vi "myo_imu_data.vi"() -> ()   [LabVIEW 2013]
uses:
  <vilib>/BLE/type_def/address_type.ctl
  type_def/unlock_types.ctl
  type_def/emg_mode.ctl
  type_def/imu_mode.ctl
  <vilib>/BLE/type_def/connection_status_bundle.ctl
panel:
  out "full message package 2":u8[](array[numeric]) format="%02x"
  out "Unlock?":bool
  out "Numeric":i32
  out "full message package":u8[][](array[numeric]) format="%02x"
  out "Battery?":bool
  out "Handler Table?":bool
  out "Connected?":bool
  out "Tank":dbl(slide) scale=0.0..100.0
  in  "stop":bool
  out "MYO Handler Table":string[][](array[string])
  out "Connection Status":T1={"MAC Address"="", "cnx handle"=0, "cnx flags"=0, "Address Type"=125, "Connection Interval (ms)"=125, "Timeout(ms)"=125, "Latency"=0, "bonding handle"=0} {"Address Type" items=["Public", "Random"]}
  in  "COM Bluegiga in":refnum<visa-resource-name>="COM13"
  out "BLED112 Dongle Info":string
  # "DONGLE"
  # "READING"
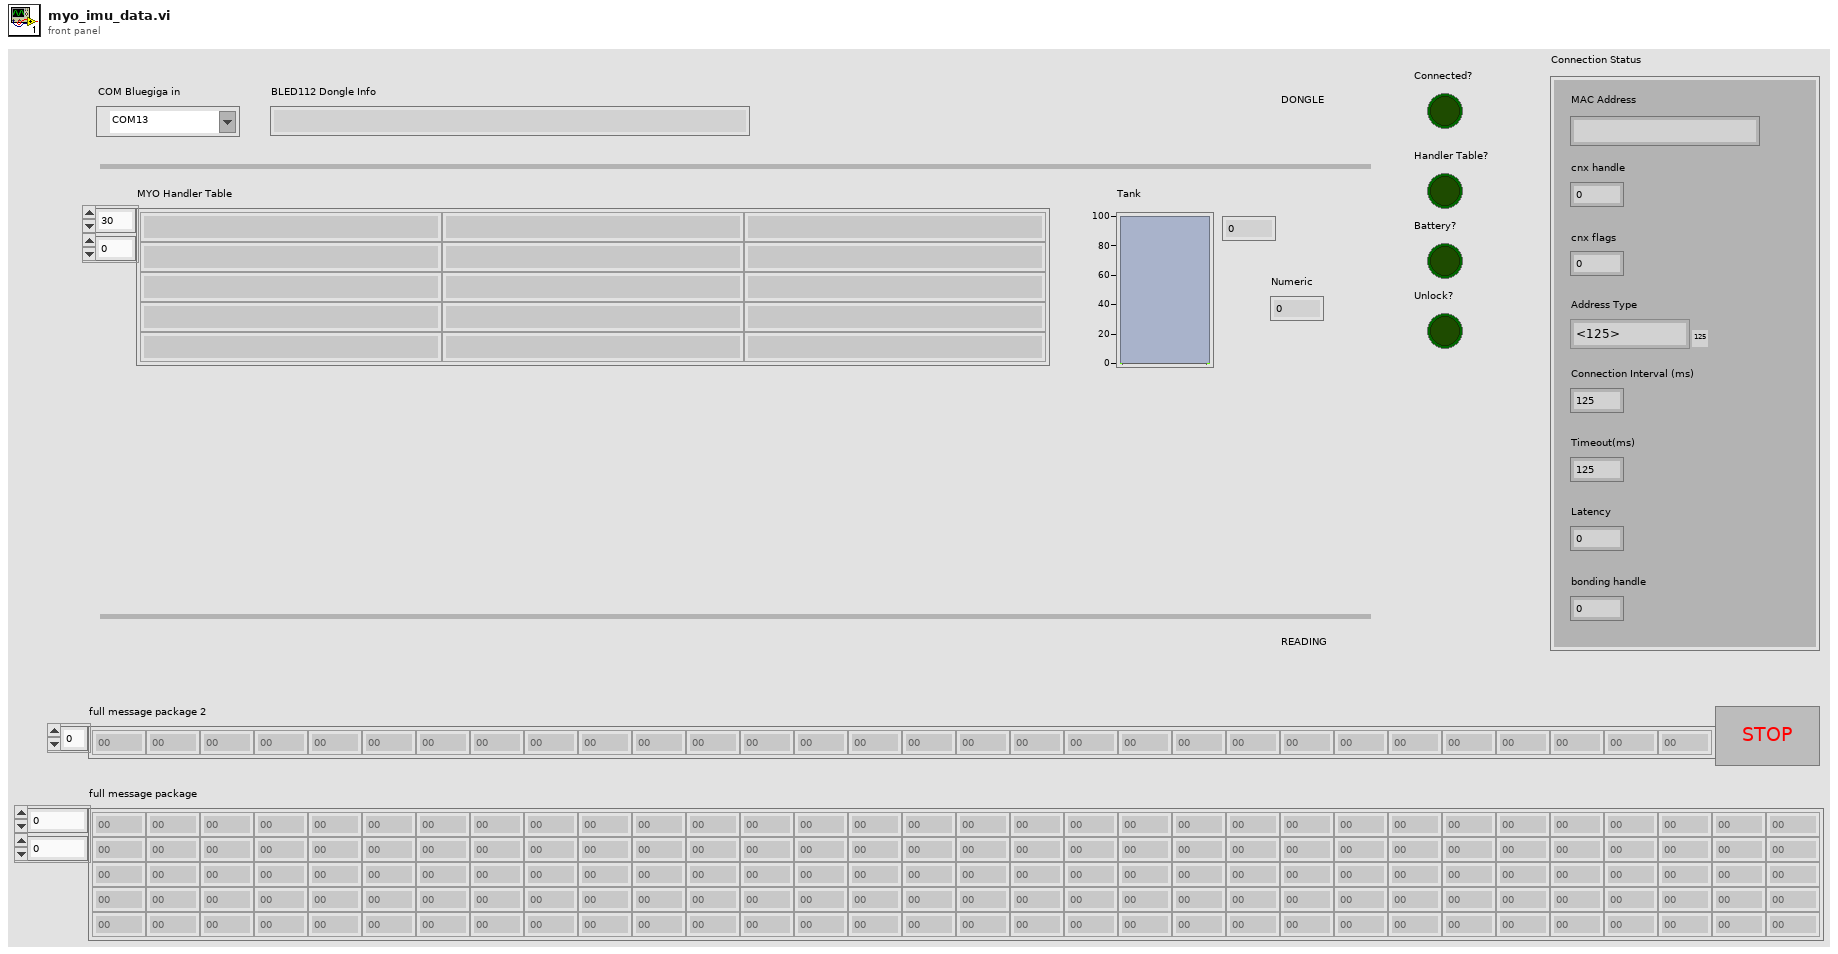
[diagram p1: front panel]
types:
  T1 = typedef "connection_status_bundle.ctl" = cluster{"MAC Address":string, "cnx handle":u8, "cnx flags":u8, "Address Type":T2, "Connection Interval (ms)":u16, "Timeout(ms)":u16, "Latency":u16, "bonding handle":u8}
  T2 = typedef "address_type.ctl" = u8
  T3 = typedef "imu_mode.ctl" = u8
  T4 = typedef "emg_mode.ctl" = u8
  T5 = typedef "unlock_types.ctl" = u8
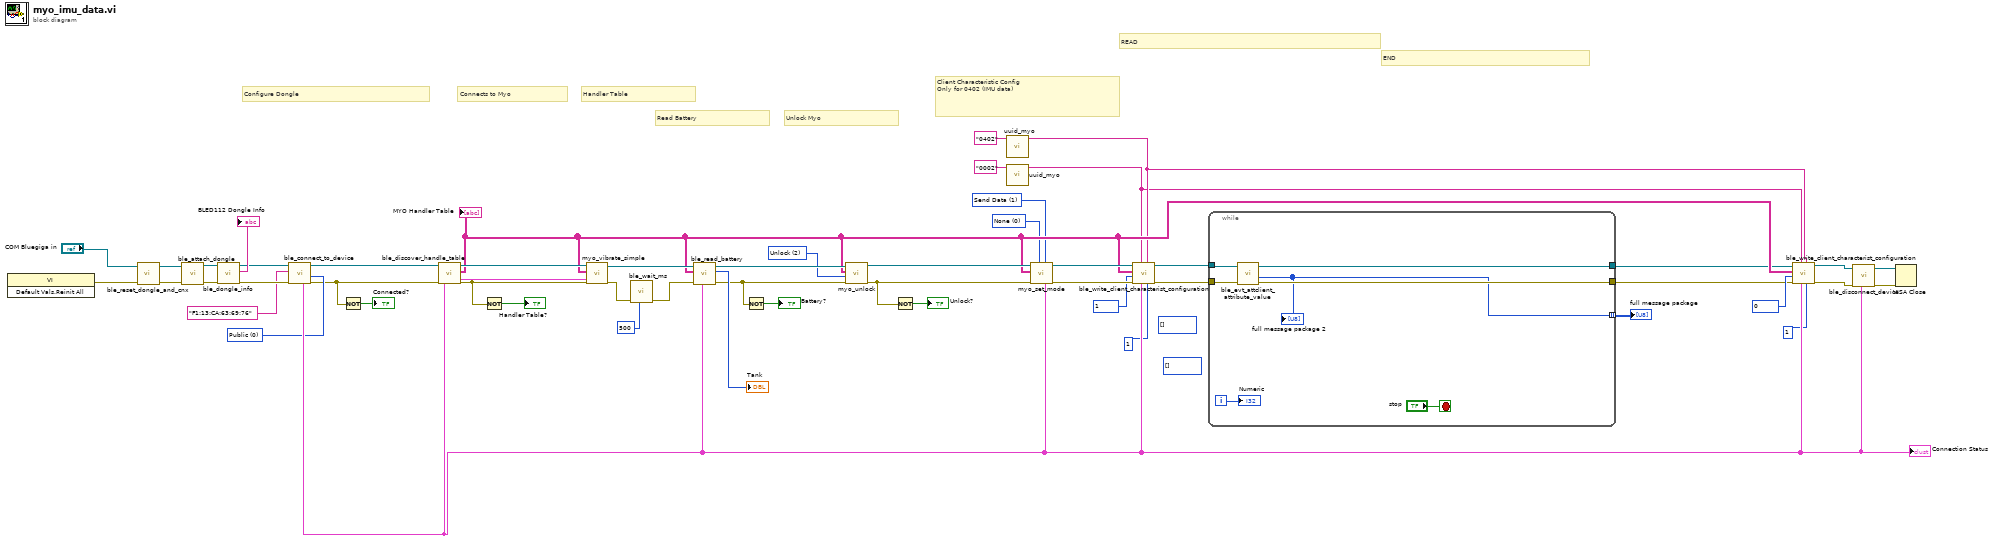
[diagram p0: block diagram]
diagram:
  w2 = T3 1 items=["None", "Send Data", "Send Events", "Send All", "Send Raw"] ("IMU mode (None)")
  (unwired) u8[] []
  (unwired) u8[] []
  w20 = T4 0 items=["None"=0, "EMG"=2, "EMG raw"=3] ("EMG mode (None)")
  w21 = T5 2 items=["Re-lock", "Unlock (timeout)", "Unlock"] ("Unlock types(Relock)")
  w37 = T2 0 items=["Public", "Random"] ("Address Type")
  # "Client Characteristic Config\nOnly for 0402 (IMU data)"
  # "Unlock Myo"
  # "Read Battery"
  # "Handler Table"
  # "Connects to Myo"
  # "END"
  # "READ"
  # "Configure Dongle"
  n1 = invoke class="VI" method="Default Vals.Reinit All"() -> (error out=w33:errorcluster)  [unwired: 3 in, 2 out]
  n2 = call <vilib>:"ble_reset_dongle_and_cnx.vi"("error in (no error)"=w33, "COM Bluegiga in"="COM Bluegiga in") -> ("error out"=w47:errorcluster, "COM Bluegiga out"=w45:refnum<visa-resource-name>)  [unwired: 8 in]
  n3 = call <vilib>:"ble_attach_dongle.vi"("error in (no error)"=w47, "COM Bluegiga in"=w45) -> ("error out"=w49:errorcluster, "COM Bluegiga out"=w48:refnum<visa-resource-name>)  [unwired: 8 in]
  n4 = call <vilib>:"ble_dongle_info.vi"("error in (no error)"=w49, "COM Bluegiga in"=w48) -> ("error out"=w40:errorcluster, "info"=→"BLED112 Dongle Info":string, "COM Bluegiga out"=w39:refnum<visa-resource-name>)  [unwired: 7 in]
  n5 = call <vilib>:"ble_connect_to_device.vi"("Address Type"=w37, "error in (no error)"=w40, "MAC Address"="F1:13:CA:63:69:76", "COM Bluegiga in"=w39) -> ("error out"=w32:errorcluster, "COM Bluegiga out"=w44:refnum<visa-resource-name>, "Connection Status"=w41:T1)  [unwired: 5 in]
  "Connection Status" <- w41
  n6 = Not(x=w32) -> (.not. x?=→"Connected?":bool)
  n7 = call <vilib>:"ble_discover_handle_table.vi"("Connection Status"=w41, "error in (no error)"=w32, "COM Bluegiga in"=w44) -> ("error out"=w30:errorcluster, "Handle table"=w22:string[][], "COM Bluegiga out"=w36:refnum<visa-resource-name>)  [unwired: 6 in]
  "MYO Handler Table" <- w22
  n8 = Not(x=w30) -> (.not. x?=→"Handler Table?":bool)
  n9 = call "myo_vibrate_simple.vi"("Connection Status"=w41, "error in (no error)"=w30, "Handle table"=w22, "VISA Refnum in"=w36) -> ("error out"=w5:errorcluster, "VISA Refnum out"=w35:refnum<visa-resource-name>)  [unwired: 6 in]
  n10 = call <vilib>:"ble_wait_ms.vi"("milliseconds to wait (100)"=u32 500, "error in (no error)"=w5) -> ("error out"=w4:errorcluster)  [unwired: 9 in]
  n11 = call <vilib>:"ble_read_battery.vi"("Connection Status"=w41, "error in (no error)"=w4, "Handle table"=w22, "VISA Refnum in"=w35) -> ("error out"=w25:errorcluster, "battery_level(%)"=→"Tank":u8, "VISA Refnum out"=w23:refnum<visa-resource-name>)  [unwired: 5 in]
  n12 = Not(x=w25) -> (.not. x?=→"Battery?":bool)
  n13 = call "myo_unlock.vi"("error in (no error)"=w25, "Unlock types(Relock)"=w21, "Handle table"=w22, "VISA Refnum in"=w23) -> ("error out"=w6:errorcluster, "VISA Refnum out"=w24:refnum<visa-resource-name>)  [unwired: 6 in]
  n14 = Not(x=w6) -> (.not. x?=→"Unlock?":bool)
  n15 = call "uuid_myo.vi"("MYO  UUID (16bits)"="0402") -> ("full UUID"=w14:string)  [unwired: 10 in]
  n16 = call "uuid_myo.vi"("MYO  UUID (16bits)"="0002") -> ("full UUID"=w12:string)  [unwired: 10 in]
  n17 = call "myo_set_mode.vi"("Connection Status"=w41, "IMU mode (None)"=w2, "EMG mode (None)"=w20, "error in (no error)"=w6, "Handle table"=w22, "VISA Refnum in"=w24) -> ("error out"=w26:errorcluster, "VISA Refnum out"=w27:refnum<visa-resource-name>)  [unwired: 4 in]
  n18 = call <vilib>:"ble_write_client_characterist_configuration.vi"(4:i16 1 ("offset"), "Characteristic UUID"=w14, "Connection Status"=w41, "Service UUID"=w12, "error in (no error)"=w26, "Value(16bit)"=u16 1, "Handle table"=w22, "COM Bluegiga in"=w27) -> ("error out"=w9:errorcluster, "COM Bluegiga out"=w10:refnum<visa-resource-name>)  [unwired: 2 in]
  n19 = while {
    tunnel: w10 -> [w58]
    tunnel: [w57] -> w17
    tunnel: [w56] -> w16
    tunnel: w9 -> [w55]
    tunnel: [w53] -> w1 mode=indexing
    i -> [w54]
    stop <- "stop" stop-if-true
    n20 = call <vilib>:"ble_evt_attclient_attribute_value.vi"("error in (no error)"=w55, "COM Bluegiga in"=w58) -> ("error out"=w56:errorcluster, "full message package"=w53:u8[], "COM Bluegiga out"=w57:refnum<visa-resource-name>)  [unwired: 6 in, 1 out]
    "full message package 2" <- w53
    "Numeric" <- w54
  }
  "full message package" <- w1
  n21 = call <vilib>:"ble_write_client_characterist_configuration.vi"(4:i16 1 ("offset"), "Characteristic UUID"=w14, "Connection Status"=w41, "Service UUID"=w12, "error in (no error)"=w16, "Value(16bit)"=u16 0, "Handle table"=w22, "COM Bluegiga in"=w17) -> ("error out"=w43:errorcluster, "COM Bluegiga out"=w42:refnum<visa-resource-name>)  [unwired: 2 in]
  n22 = call <vilib>:"ble_disconnect_device.vi"("Connection Status"=w41, "error in (no error)"=w43, "COM Bluegiga in"=w42) -> ("error out"=w50:errorcluster, "COM Bluegiga out"=w51:refnum<visa-resource-name>)  [unwired: 7 in]
  n23 = VISA Close(VISA resource name=w51, error in (no error)=w50) -> ()  [unwired: 1 out]
